vi "CheckCollision.vi"(8 "error in":errorcluster, 10 "sprite in":refnum<class "Sprite.lvclass">, 11 "class data in":refnum<class "Brick.lvclass">) -> (0 "error out":errorcluster, 1 "collisionInfo out":cluster{"collision":bool, "fatal":bool}, 2 "sprite out":refnum<class "Sprite.lvclass">, 3 "class data out":refnum<class "Brick.lvclass">)   [LabVIEW 2010, in "Labricks.lvlib" / "Brick.lvclass"]
uses:
  Brick.lvclass
  RenderBase/Sprite_class/Sprite.lvclass
  RenderBase/SceneRoot_class/SceneRoot.lvclass
  RenderBase/SceneObject_class/properties/SceneRoot/GetSceneRoot.vi
  RenderBase/SceneObject_class/properties/Position/GetPosition.vi
  Game_class/Game.lvclass
  <vilib>/picture/3D Picture Control/NI_3D Picture Control.lvlib
  RenderBase/SceneObject_class/SceneObject.lvclass
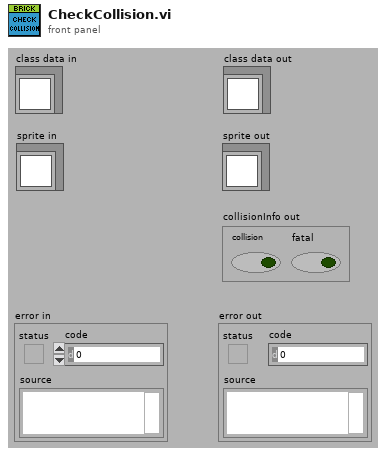
[diagram p1: front panel]
types:
  T1 = typedef "LV3DPointTypeDef.ctl" = cluster{"X":sgl, "Y":sgl, "Z":sgl}
  T2 = typedef "RenderBase.lvlib/SceneObject.lvclass/CollisionAction.ctl" = enum16{"None", "BounceX", "BounceY", "BounceXY"}
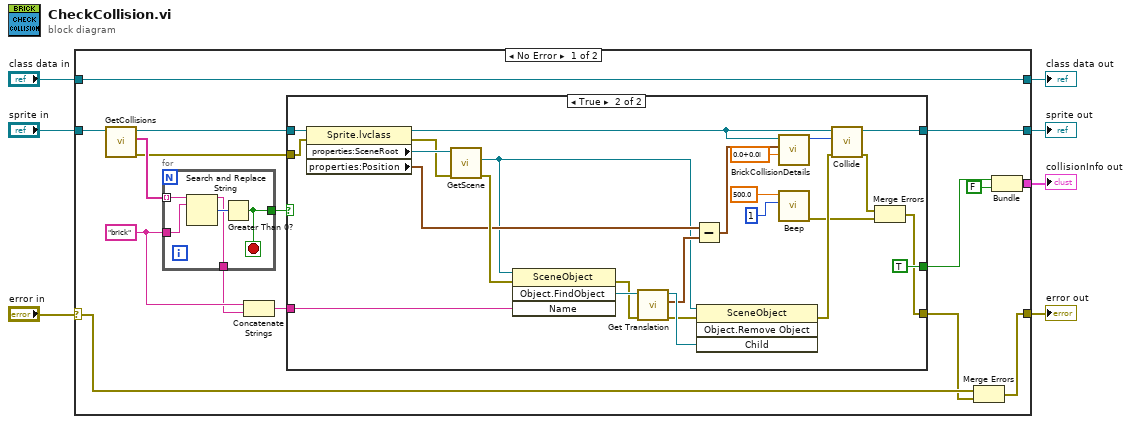
[diagram p0: block diagram]
diagram:
  n1 = case shown="No Error" "error in" {
    selector: "error in" -> [w20 w58]
    tunnel: [w21 w58] -> w7
    tunnel: "sprite in" -> [w14 w56]
    tunnel: [w23 w57] -> w5
    tunnel: "class data in" -> [w23 w57]
    tunnel: [w17 w56] -> w2
    tunnel: [w19 _] -> w1
    frame No Error {
      w10 = "brick" ("search string")
      n2 = call-dynamic "GetCollisions.vi"("sprite in"=w14) -> ("error out"=w11:errorcluster, "collisions out"=w13:string[], "sprite out"=w15:refnum<class "Sprite.lvclass">)  [unwired: 8 in]
      n3 = for {
        tunnel: w13 -> [w27] mode=indexing
        tunnel: w10 -> [w26]
        tunnel: [w25] -> w12
        tunnel: [w24] -> w8
        stop <- w25 stop-if-true
        n4 = Search and Replace String(input string=w27, search string=w26) -> (result string=w24:string, number of replacements=w28:i32)  [unwired: 6 in, 2 out]
        n5 = Greater Than 0?(x=w28) -> (x > 0?=w25:bool)
      }
      n6 = Concatenate Strings(w10, w8) -> (w9:string)
      n7 = case shown="True" w12 {
        tunnel: [w29 w46] -> w16
        tunnel: [_ TRUE] -> w22
        tunnel: w15 -> [w30 w38]
        tunnel: [w30 w49] -> w17
        tunnel: w11 -> [w29 w37]
        tunnel: w9 -> [_ w34]
        frame False {
        }
        frame True {
          n8 = property class="Sprite.lvclass"(reference=w38, error in=w37) -> (reference out=w36:refnum<class "Sprite.lvclass">, error out=w40:errorcluster, "properties:SceneRoot"=w41:refnum<class "SceneRoot.lvclass">, "properties:Position"=w35:T1)
          n9 = call "GetScene.vi"("error in (no error)"=w40, "reference in"=w41) -> ("error out"=w39:errorcluster, "Scene"=w31:refnum<vi>)  [unwired: 7 in, 1 out]
          n10 = invoke class="SceneObject" method="Object.FindObject"(reference=w31, error in=w39, "Name"=w34) -> (error out=w32:errorcluster, "FindObject"=w33:refnum<vi>)  [unwired: 1 in, 2 out]
          n11 = call <vilib>:"Get Translation.vi"("error in (no error)"=w32, "Scene Object"=w33) -> ("error out"=w51:errorcluster, "Transformation:Get Translation"=w50:cluster{"X":sgl, "Y":sgl, "Z":sgl}, "Scene Object"=w52:refnum<vi>)  [unwired: 7 in]
          n12 = Subtract(x=w35, y=w50) -> (x-y=w44:T1)
          n13 = invoke class="SceneObject" method="Object.Remove Object"(reference=w31, error in=w51, "Child"=w52) -> (error out=w47:errorcluster)  [unwired: 1 in, 3 out]
          n14 = call "BrickCollisionDetails.vi"("direction in"=cdb 0.0+0.0i, "position in"=w44, "class data in"=w36) -> ("collisionAction out"=w43:T2)  [unwired: 8 in]
          n15 = call "Beep.vi"("numChunks in"=1 ("#s"), "frequency in"=500.0 ("frequency")) -> ("error out"=w45:errorcluster)  [unwired: 9 in]
          n16 = call-dynamic "Collide.vi"("error in (no error)"=w47, "action in"=w43, "class data in"=w36) -> ("error out"=w48:errorcluster, "class data out"=w49:refnum<class "Sprite.lvclass">)  [unwired: 7 in]
          n17 = Merge Errors(w48, w45) -> (w46:errorcluster)
        }
      }
      n18 = Merge Errors(w20, w16) -> (w21:errorcluster)
      n19 = Bundle(w22, FALSE) -> (w19:cluster{bool, bool})  [unwired: 1 in]
    }
    frame Error {
    }
  }
  "error out" <- w7
  "class data out" <- w5
  "sprite out" <- w2
  "collisionInfo out" <- w1
